vi "serial_send.vi"(8 "error in (no error)":errorcluster, 10 "Send buffer":string, 11 "VISA in":refnum<visa-resource-name>) -> (0 "error out":errorcluster, 3 "VISA out":refnum<visa-resource-name>)   [LabVIEW 2022 SP3]
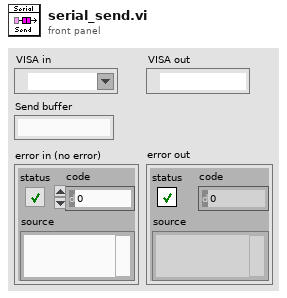
[diagram p1: front panel]
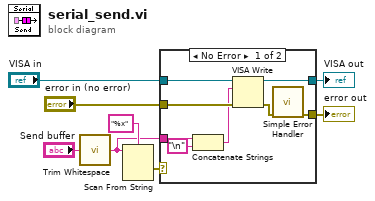
[diagram p0: block diagram]
diagram:
  n1 = call <vilib>:"Trim Whitespace.vi"("string"="Send buffer") -> ("trimmed string"=w1:string)  [unwired: 1 in]
  n2 = Scan From String(format string="%x", input string=w1) -> (error out=w2:errorcluster)  [unwired: 4 in, 2 out]
  n3 = case shown="No Error" w2 {
    tunnel: [w14 w17] -> w8
    tunnel: "VISA in" -> [w13 w17]
    tunnel: "error in (no error)" -> [w12 w18]
    tunnel: [w10 w18] -> w5
    tunnel: w1 -> [w9 _]
    frame No Error {
      n4 = Concatenate Strings(w9, "\n") -> (w11:string)
      n5 = VISA Write(VISA resource name=w13, write buffer=w11, error in (no error)=w12) -> (VISA resource name out=w14:refnum<visa-resource-name>, error out=w15:errorcluster)  [unwired: 1 out]
      n6 = call <vilib>:"Simple Error Handler.vi"("error in (no error)"=w15) -> ("error out"=w10:errorcluster)  [unwired: 4 in, 4 out]
    }
    frame Error {
    }
  }
  "VISA out" <- w8
  "error out" <- w5
